vi "AD7747_Calibration.vi"(8 "error in":errorcluster, 10 "Read After CapDac?":bool, 11 "Cap_Dac Value":u8=139 format="%.0x") -> (0 "errorout":errorcluster, 3 "AD7747 Values":string[][](table))   [LabVIEW 2012]
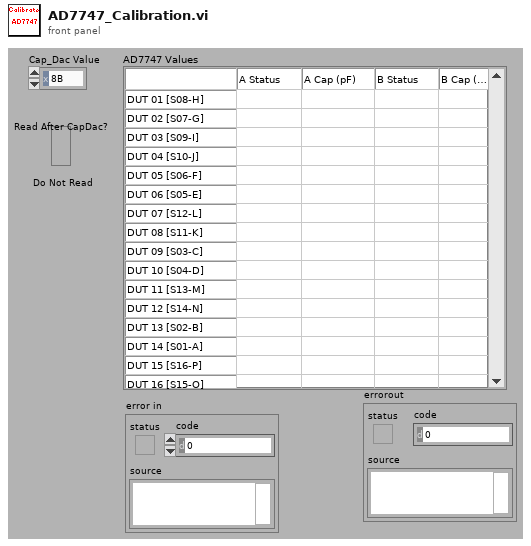
[diagram p1: front panel]
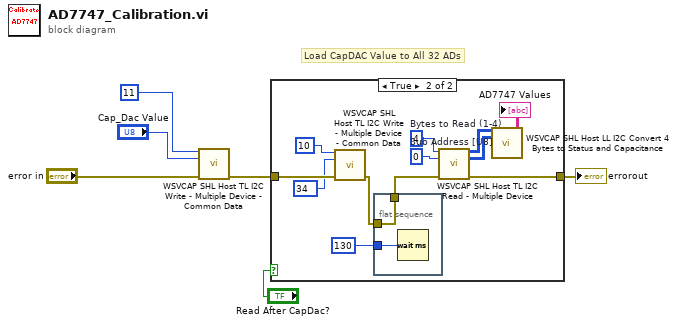
[diagram p0: block diagram]
diagram:
  # "Load CapDAC Value to All 32 ADs"
  n1 = call "WSVCAP SHL Host TL I2C Write - Multiple Device - Common Data.vi"("Sub Address"=u8 11, "Data Out [U8]"="Cap_Dac Value", "error in"="error in") -> ("error out"=w2:errorcluster)  [unwired: 12 in]
  n2 = case shown="True" "Read After CapDac?" {
    tunnel: w2 -> [w7 w13]
    tunnel: [w7 w14] -> w1
    frame False {
    }
    frame True {
      w18 = u8 4  # Bytes to Read (1-4)
      w19 = u8 0  # Sub Address [U8]
      n3 = call "WSVCAP SHL Host TL I2C Write - Multiple Device - Common Data.vi"("Sub Address"=u8 10, "Data Out [U8]"=u8 34 ("Sub Address"), "error in"=w13) -> ("error out"=w10:errorcluster)  [unwired: 12 in]
      n4 = flat-sequence {
        tunnel: w10 -> [w21]
        tunnel: [w21] -> w9
        tunnel: u32 130 ("milliseconds to wait") -> [w20]
        frame #0 {
          n5 = Wait (ms)(milliseconds to wait=w20) -> ()  [unwired: 1 out]
        }
      }
      n6 = call "WSVCAP SHL Host TL I2C Read - Multiple Device.vi"("Bytes to Read (1-4)"=w18, "Sub Address [U8]"=w19, "error in"=w9) -> ("A1-A16 Read Data [U8]"=w17:u8[][], "B1-B16 Read Data [U8]"=w16:u8[][], "error out"=w14:errorcluster)  [unwired: 10 in]
      n7 = call "WSVCAP SHL Host LL I2C Convert 4 Bytes to Status and Capacitance.vi"("A1-A16 Read Data [U8]"=w17, "B1-B16 Read Data [U8]"=w16) -> ("AD7747 Values"=→"AD7747 Values":string[][])  [unwired: 13 in]
    }
  }
  "errorout" <- w1
